vi "onStart.vi"(8 "error in (no error)":errorcluster, 11 "MAUI":refnum<class "MAUI.lvclass">) -> (0 "error out":errorcluster, 3 "MAUI out":refnum<class "MAUI.lvclass">)   [LabVIEW 2016, in "MAUI.lvclass"]
doc: "JKI State Machine Objects (SMO) 1.3.0.56\nJKI - JKI\nCopyright (c) 2017, JKI"
uses:
  MAUI.lvclass
  <vilib>/Levylab/Embedded SMO UI/EmbeddedSMO.lvclass
  C:/Program Files (x86)/National Instruments/LabVIEW 2016/vi.lib/JKI/JKI SMO/SMO/SMO.lvclass
  MAUI.lvclass/MAUI.ctl
  <vilib>/JKI/JKI SMO/SMO.UI/SMO.UI.lvclass
  <vilib>/JKI/JKI SMO/SMO/SMO.lvclass
panel:
  # "For instructions on how to use the JKI State Machine Objects, examples and video tutorials, visit:\nhttp://jki.net/state-machine-objects/\n\nJKI State Machine Objects™\nhttp://jki.net/state-machine-objects/\nCopyright (C) 2005-2015, JKI <info@jki.net>\nALL RIGHTS RESERVED"
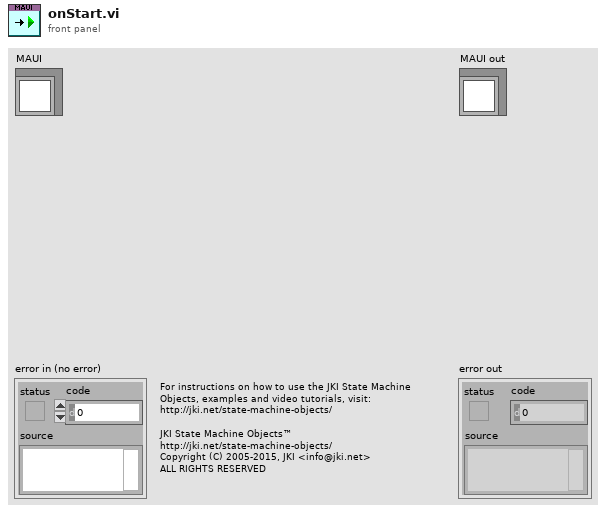
[diagram p1: front panel]
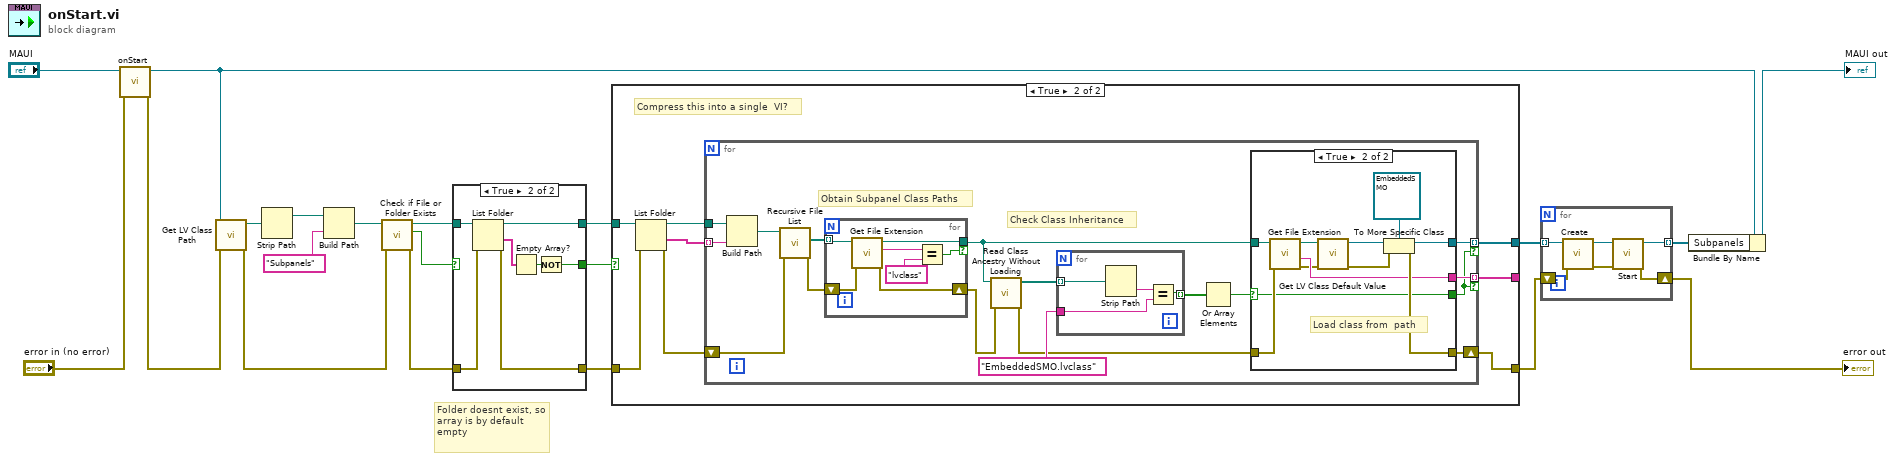
[diagram p0: block diagram]
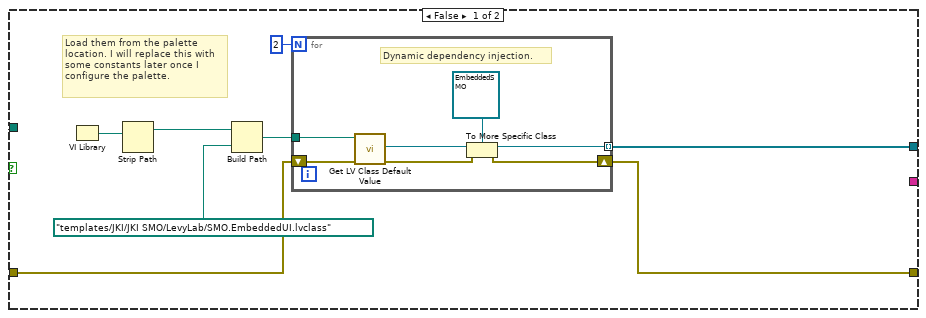
[diagram p3: hidden frame]
diagram:
  # "Folder doesnt exist, so array is by default empty"
  n1 = call-parent "onStart.vi"("error in (no error)"="error in (no error)", "SMO"="MAUI") -> ("error out"=w15:errorcluster, "SMO out"=w9:refnum<class "MAUI.lvclass">)  [unwired: 8 in]
  n2 = call <vilib>:"Get LV Class Path.vi"("error in (no error)"=w15, "object"=w9) -> ("error out"=w16:errorcluster, "class path"=w20:path)  [unwired: 8 in]
  n3 = Strip Path(path=w20) -> (stripped path=w19:path)  [unwired: 1 out]
  n4 = Build Path(base path=w19, name or relative path="Subpanels") -> (appended path=w17:path)
  n5 = call <vilib>:"Check if File or Folder Exists.vi"("error in (no error)"=w16, "path"=w17) -> ("error out"=w6:errorcluster, "file or folder exists?"=w5:bool, "dup path"=w8:path)  [unwired: 7 in]
  n6 = case shown="True" w5 {
    selector: w5 -> [w21 _]
    tunnel: w8 -> [w23 w30]
    tunnel: [w23 w29] -> w7
    tunnel: w6 -> [w22 w28]
    tunnel: [w22 w27] -> w4
    tunnel: [w21 w25] -> w1
    frame False {
    }
    frame True {
      n7 = List Folder(path=w30, error in=w28) -> (path out=w29:path, folder names=w24:string[], error out=w27:errorcluster)  [unwired: 2 in, 1 out]
      n8 = Empty Array?(array=w24) -> (empty?=w26:bool)
      n9 = Not(x=w26) -> (.not. x?=w25:bool)
    }
  }
  n10 = case shown="True" w1 {
    tunnel: w7 -> [w39 w54]
    tunnel: w4 -> [w35 w49]
    tunnel: [w33 w48] -> w3
    tunnel: [w31 w50] -> w14
    tunnel: [_ w47] -> _
    frame False {
      # "Load them from the palette location. I will replace this with some constants later once I configure the palette."
      n11 = Create Folder(path (use dialog)=w39, error in=w35) -> ()  [unwired: 1 in, 3 out]
      n12 = VI Library() -> (path=w38:path)
      n13 = Strip Path(path=w38) -> (stripped path=w37:path)  [unwired: 1 out]
      n14 = Build Path(base path=w37, name or relative path=path "templates/JKI/JKI SMO/LevyLab/SMO.EmbeddedUI.lvclass") -> (appended path=w32:path)
      n15 = for {
        N: 2 -> [_]
        tunnel: w32 -> [w46]
        shift-right: [w41] -> w33
        shift-left: w35 -> [w45]
        tunnel: [w42] -> w31 mode=indexing
        # "Dynamic dependency injection."
        n16 = call <vilib>:"Get LV Class Default Value.vi"("error in (no error)"=w45, "class path"=w46) -> ("error out"=w40:errorcluster, "object"=w44:refnum<class>)  [unwired: 8 in]
        n17 = To More Specific Class(target class=refnum<class "EmbeddedSMO.lvclass"> refnum ("EmbeddedSMO"), reference=w44, error in=w40) -> (specific class reference=w42:refnum<class "EmbeddedSMO.lvclass">, error out=w41:errorcluster)
      }
    }
    frame True {
      # "Compress this into a single  VI?"
      n18 = List Folder(path=w54, error in=w49) -> (path out=w53:path, folder names=w52:string[], error out=w51:errorcluster)  [unwired: 2 in, 1 out]
      n19 = for {
        tunnel: w53 -> [w71]
        tunnel: w52 -> [w70] mode=indexing
        tunnel: [w66] -> w50 mode=indexing if=w55
        shift-right: [w58] -> w48
        shift-left: w51 -> [w62]
        tunnel: [w56] -> w47 mode=indexing if=w55
        # "Check Class Inheritance"
        # "Obtain Subpanel Class Paths"
        n20 = Build Path(base path=w71, name or relative path=w70) -> (appended path=w69:path)
        n21 = call <vilib>:"Recursive File List.vi"("error in (no error)"=w62, "Folder Path"=w69) -> ("error out"=w61:errorcluster, "All Files in Dir"=w68:path[])  [unwired: 5 in, 3 out]
        n22 = for {
          tunnel: w68 -> [w93] mode=indexing
          tunnel: [w92] -> w67 if=w91
          shift-right: [w89] -> w60
          shift-left: w61 -> [w90]
          n23 = call <vilib>:"Get File Extension.vi"("error in (no error)"=w90, "file"=w93) -> ("error out"=w89:errorcluster, "lowercase file extension"=w95:string, "dup file"=w92:path)  [unwired: 5 in, 2 out]
          n24 = Equal?(x=w95, y="lvclass") -> (x = y?=w91:bool)
        }
        n25 = call <vilib>:"Read Class Ancestry Without Loading.vi"("error in (no error)"=w60, "LabVIEW Class Path"=w67) -> ("error out"=w59:errorcluster, "Class Ancestry"=w65:path[])  [unwired: 8 in]
        n26 = for {
          tunnel: w65 -> [w88] mode=indexing
          tunnel: [w86] -> w64 mode=indexing
          tunnel: "EmbeddedSMO.lvclass" -> [w85]
          n27 = Strip Path(path=w88) -> (name=w87:string)  [unwired: 1 out]
          n28 = Equal?(x=w87, y=w85) -> (x = y?=w86:bool)
        }
        n29 = Or Array Elements(Boolean array=w64) -> (logical OR=w57:bool)
        n30 = case shown="True" w57 {
          selector: w57 -> [w72 w74]
          tunnel: w67 -> [_ w79]
          tunnel: [_ w84] -> w66
          tunnel: w59 -> [w73 w76]
          tunnel: [w73 w80] -> w58
          tunnel: [_ w77] -> w56
          tunnel: [w72 w74] -> w55
          frame False {
            # "This case gets filtered later by conditional terminals. Don't do anything here."
            # "This case gets filtered later by conditional terminals"
          }
          frame True {
            # "Load class from  path"
            n31 = call <vilib>:"Get File Extension.vi"("error in (no error)"=w76, "file"=w79) -> ("error out"=w75:errorcluster, "filename without extension"=w77:string, "dup file"=w78:path)  [unwired: 5 in, 2 out]
            n32 = call <vilib>:"Get LV Class Default Value.vi"("error in (no error)"=w75, "class path"=w78) -> ("error out"=w81:errorcluster, "object"=w83:refnum<class>)  [unwired: 8 in]
            n33 = To More Specific Class(target class=refnum<class "EmbeddedSMO.lvclass"> refnum ("EmbeddedSMO"), reference=w83, error in=w81) -> (specific class reference=w84:refnum<class "EmbeddedSMO.lvclass">, error out=w80:errorcluster)
          }
        }
      }
    }
  }
  n34 = for {
    tunnel: w14 -> [w101] mode=indexing
    tunnel: [w100] -> w10 mode=indexing
    shift-right: [w96] -> w11
    shift-left: w3 -> [w97]
    n35 = call <vilib>:"Create.vi"("error in (no error)"=w97, "SMO"=w101) -> ("error out"=w98:errorcluster, "SMO out"=w99:refnum<class "EmbeddedSMO.lvclass">)  [unwired: 7 in, 1 out]
    n36 = call <vilib>:"Start.vi"("error in (no error)"=w98, "SMO"=w99) -> ("error out"=w96:errorcluster, "SMO out"=w100:refnum<class "EmbeddedSMO.lvclass">)  [unwired: 8 in]
  }
  "error out" <- w11
  n37 = Bundle By Name(cluster=w9, "Subpanels"=w10) -> (→"MAUI out":refnum<class "MAUI.lvclass">)
